vi "Stop Flush Message.vi"(8 "error in (no error)":errorcluster, 11 "Report Generator in":refnum<class "Report Generator.lvclass">) -> (0 "error out":errorcluster, 3 "Report Generator out":refnum<class "Report Generator.lvclass">)   [LabVIEW 2023, in "Report Generator.lvlib" / "Report Generator.lvclass"]
uses:
  Library/Report Generator.lvclass
  Library/Report Generator.lvclass/Report Generator.ctl
  builds/Engine/Actor Framework.lvlibp/1abvi3w/vi.lib/ActorFramework/Time-Delayed Send Message/Time-Delay Override Options.ctl
  builds/Engine/Actor Framework.lvlibp
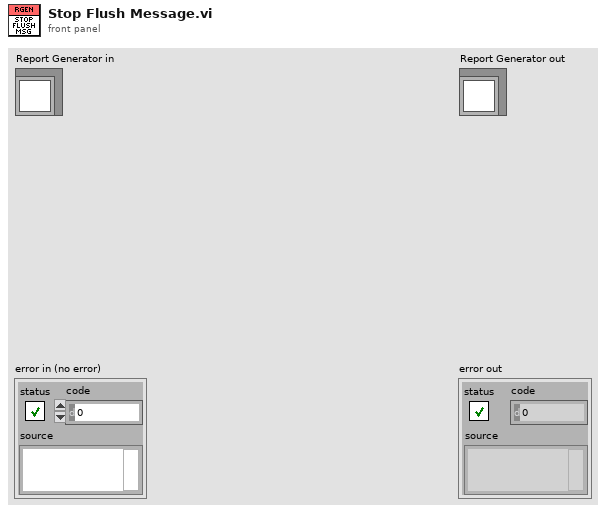
[diagram p1: front panel]
types:
  T1 = typedef "Actor Framework.lvlibp/Time-Delay Override Options.ctl" = enum16{"Send next copy now", "Skip next scheduled copy", "Send next copy now and stop all further copies", "Stop all further copies"}
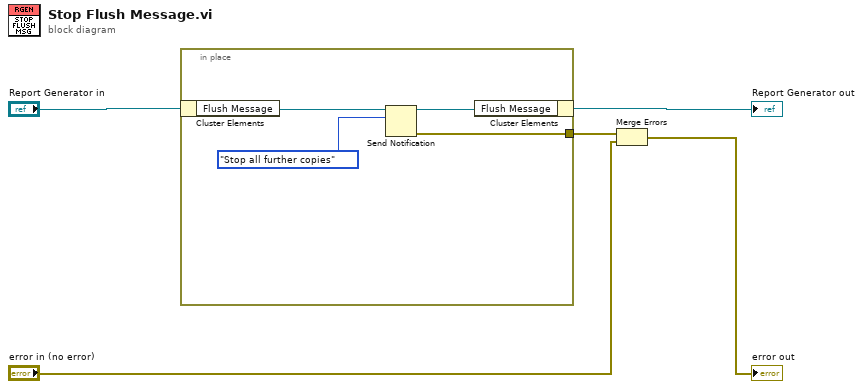
[diagram p0: block diagram]
diagram:
  n1 = in-place {
    in-place-border: [w6] -> w3
    n2 = in-place-cluster #1("Report Generator in") -> ("Flush Message"=w9:refnum<notifier>)
    n3 = Send Notification(notification=Time-Delay_Override_Options."Stop all further copies", notifier=w9) -> (notifier out=w8:refnum<notifier>, error out=w6:errorcluster)  [unwired: 1 in]
    n4 = in-place-cluster #1("Flush Message"=w8) -> (→"Report Generator out":refnum<class "Report Generator.lvclass">)
  }
  n5 = Merge Errors(w3, "error in (no error)") -> (→"error out":errorcluster)
